vi "Enabled-Disabled.vi"(11 "Tons of Peanuts":i8) -> (1 "Tons of Peanuts":i8, 2 "Use Peanuts Control Status":T1(ring), 3 "Fill Peanuts Control Status":T1(ring))   [LabVIEW 2020]
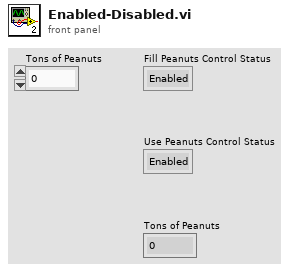
[diagram p1: front panel]
types:
  T1 = enum8{"Enabled", "Disabled", "Disabled and Grayed Out"}
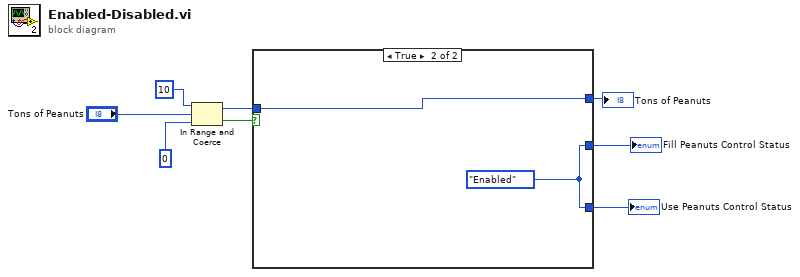
[diagram p0: block diagram]
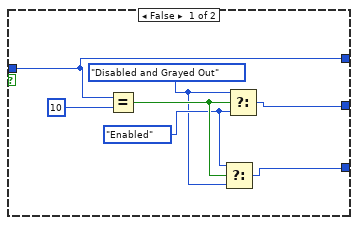
[diagram p2: hidden frame]
diagram:
  n1 = In Range and Coerce(upper limit=i8 10, x="Tons of Peanuts", lower limit=i8 0) -> (coerced(x)=w5:i8, In Range?=w4:bool)
  n2 = case shown="True" w4 {
    tunnel: w5 -> [w9 w16]
    tunnel: [w11 w17] -> w7
    tunnel: [w10 w17] -> w8
    tunnel: [w9 w16] -> w1
    frame False {
      w13 = T1."Enabled" ("Disabled")
      w12 = T1."Disabled and Grayed Out" ("Disabled")
      n3 = Equal?(x=w9, y=i8 10) -> (x = y?=w14:bool)
      n4 = Select(t=w13, s=w14, f=w12) -> (s? t:f=w10:T1)
      n5 = Select(t=w12, s=w14, f=w13) -> (s? t:f=w11:T1)
    }
    frame True {
      w17 = T1."Enabled" ("Disabled")
    }
  }
  "Use Peanuts Control Status" <- w8
  "Fill Peanuts Control Status" <- w7
  "Tons of Peanuts" <- w1
